vi "PID Single.vi"(7 "initialize":bool, 8 "Limits":cluster{"output high":dbl, "output low":dbl}, 9 "PID gains in":T1, 10 "Variable":dbl, 11 "Setpoint":dbl) -> (3 "Out":dbl)   [LabVIEW 2018]
uses:
  <vilib>/ptbypt/NI_PtbyPt.lvlib
panel:
  out "Waveform Chart 2":dbl[][](graph)
  out "Waveform Chart":dbl[][](graph)
  out "PID Values":dbl[](array[numeric])
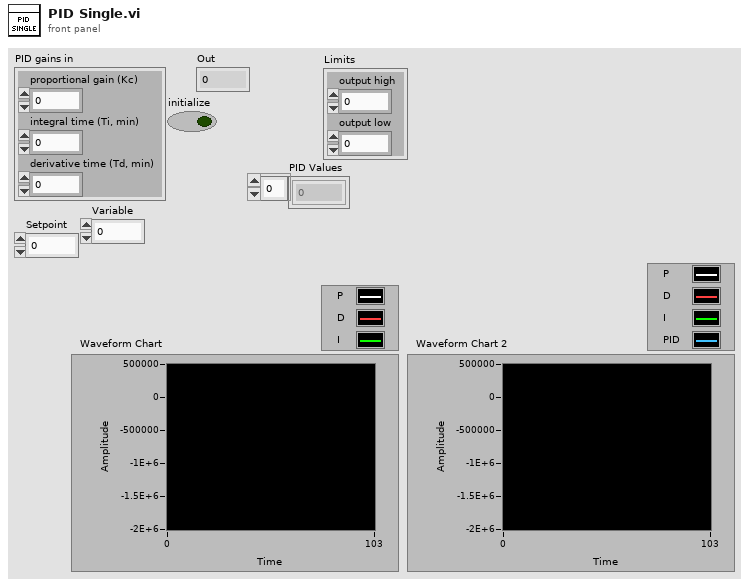
[diagram p1: front panel]
types:
  T1 = cluster{"proportional gain (Kc)":dbl, "integral time (Ti, min)":dbl, "derivative time (Td, min)":dbl}
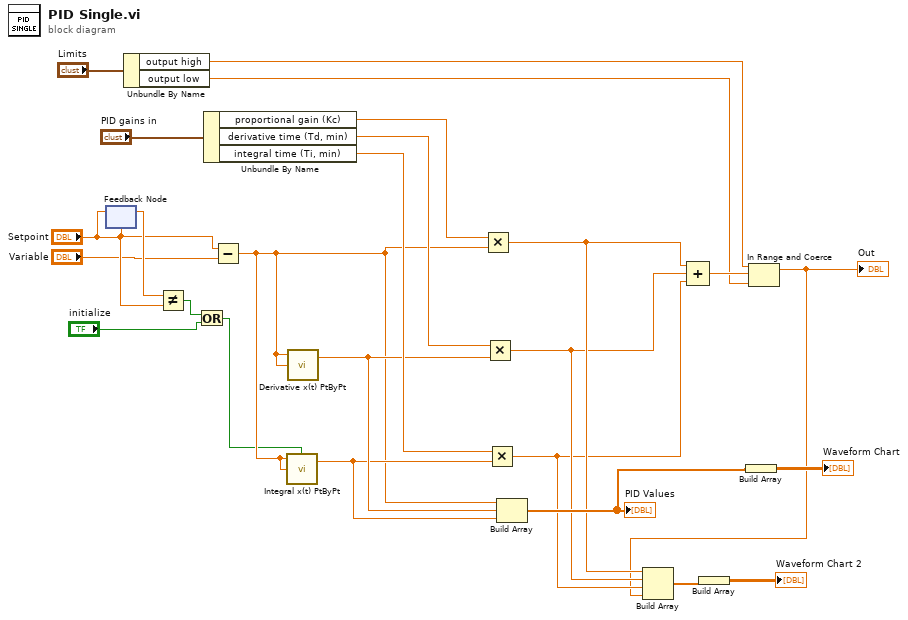
[diagram p0: block diagram]
diagram:
  n1 = feedback-in #1("Setpoint") -> ()
  n2 = feedback #1("Setpoint") -> (w21:dbl)
  n3 = Unbundle By Name("Limits") -> ("output high"=w12:dbl, "output low"=w11:dbl)
  n4 = Not Equal?(x=w21, y="Setpoint") -> (x != y?=w22:bool)
  n5 = Or(x=w22, y="initialize") -> (x .or. y?=w7:bool)
  n6 = Unbundle By Name("PID gains in") -> ("proportional gain (Kc)"=w18:dbl, "derivative time (Td, min)"=w17:dbl, "integral time (Ti, min)"=w16:dbl)
  n7 = Subtract(x="Setpoint", y="Variable") -> (x-y=w8:dbl)
  n8 = call <vilib>:"Integral x(t) PtByPt.vi"("initialize"=w7, "initial condition"=w8, "x"=w8) -> ("integral x(t)"=w14:dbl)  [unwired: 1 in, 1 out]
  n9 = call <vilib>:"Derivative x(t) PtByPt.vi"("initial condition"=w8, "x"=w8) -> ("dx/dt"=w15:dbl)  [unwired: 2 in, 1 out]
  n10 = Multiply(x=w18, y=w8) -> (x*y=w5:dbl)
  n11 = Multiply(x=w17, y=w15) -> (x*y=w4:dbl)
  n12 = Multiply(x=w16, y=w14) -> (x*y=w3:dbl)
  n13 = Build Array(w8, w15, w14) -> (w20:dbl[])
  "PID Values" <- w20
  n14 = Compound Arithmetic op=ADD(w5, w4, w3) -> (w13:dbl)
  n15 = Build Array(w20) -> (→"Waveform Chart":dbl[][])
  n16 = In Range and Coerce(upper limit=w12, x=w13, lower limit=w11) -> (coerced(x)=w2:dbl)  [unwired: 1 out]
  "Out" <- w2
  n17 = Build Array(w5, w4, w3, w2) -> (w6:dbl[])
  n18 = Build Array(w6) -> (→"Waveform Chart 2":dbl[][])
